vi "subscribe.vi"(8 "Error In":errorcluster, 10 "qos (1)":i32=1, 11 "topic (test/#)":string="test/#") -> (0 "Error Out":errorcluster)   [LabVIEW 2016, in "mqtt.lvlib"]
uses:
  mqtt.lvlib
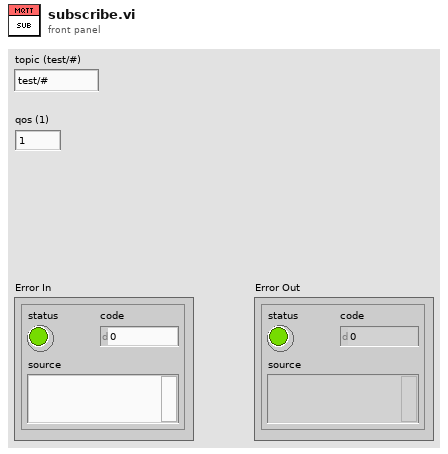
[diagram p1: front panel]
types:
  T1 = enum16{"big-endian, network order", "native, host order", "little-endian"}
  T2 = cluster{"command":string, "topic":string, "qos":i32}
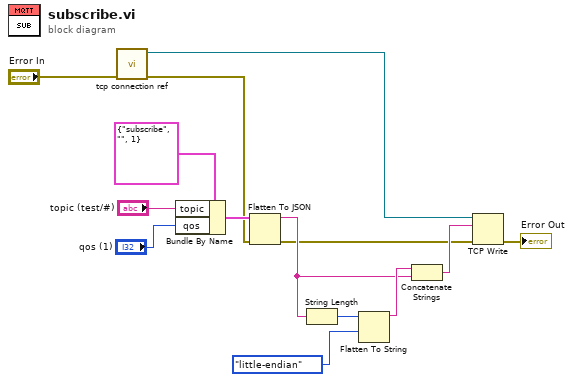
[diagram p0: block diagram]
diagram:
  n1 = call "tcp connection ref.vi"("Error In"="Error In") -> ("Error Out"=w4:errorcluster, "tcpRef"=w2:refnum<k5>)  [unwired: 9 in]
  n2 = Bundle By Name(cluster=T2 {"command"="subscribe", "topic"="", "qos"=1} ("subscribe"), "topic"="topic (test/#)", "qos"="qos (1)") -> (w7:T2)
  n3 = Flatten To JSON(anything=w7, error in (no error)=w4) -> (JSON string=w6:string, 11:w3:errorcluster)  [unwired: 1 in]
  n4 = String Length(string=w6) -> (length=w10:i32)
  n5 = Flatten To String(anything=w10, byte order (0:big-endian, network order)=T1."little-endian") -> (data string=w9:string)  [unwired: 2 in, 2 out]
  n6 = Concatenate Strings(w9, w6) -> (w8:string)
  n7 = TCP Write(connection ID=w2, data in=w8, error in (no error)=w3) -> (error out=→"Error Out":errorcluster)  [unwired: 1 in, 2 out]
